vi "Get Channel Groups.vi"(7 "Settings(JSON)":string, 8 "error in":errorcluster, 9 "Channel Paths":string[](array[string]), 10 "Channel TypeNames":string[](array[string]), 11 "Channel JSONs":string[](array[string])) -> (0 "error out":errorcluster, 3 "ChannelGroups":T1, 5 "Settings(JSON)":string)   [LabVIEW 2026, in "Template Deployment Hooks.lvlib"]
uses:
  Template Deployment Hooks.lvlib
  Types/Channel Mode.ctl
  <vilib>/JDP Science/JSONtext/Next JSON Value.vi
  <vilib>/JDP Science/JSONtext/String Subset.vi
  <vilib>/JDP Science/JSONtext/support/Strip Quotes and Unescape.vi
  <vilib>/JDP Science/JSONtext/Parsing/Advance past next JSON Value (inlined COPY).vi
  <vilib>/JDP Science/JSONtext/support/Unescape JSON string.vi
  <vilib>/JDP Science/JSONtext/Parsing/Advance past whitespace.vi
  <vilib>/JDP Science/JSONtext/Parsing/Advance past String.vi
  <vilib>/JDP Science/JSONtext/Parsing/Advance past Number.vi
  <vilib>/JDP Science/JSONtext/Parsing/Advance past Line Ending.vi
  <vilib>/JDP Science/JSONtext/Parsing/Parse Full Path or Item Name.vi
  <vilib>/JDP Science/JSONtext/Parsing/Advance past Array.vi
  <vilib>/JDP Science/JSONtext/Parsing/Advance past Object.vi
  <vilib>/JDP Science/JSONtext/support/Error Cluster From Code.vi
  <vilib>/JDP Science/JSONtext/Offset/Find Item Locations by Path.vi
  <vilib>/JDP Science/JSONtext/Parsing/Advance past next JSON Value.vi
  <vilib>/JDP Science/JSONtext/JSONtext.lvlib
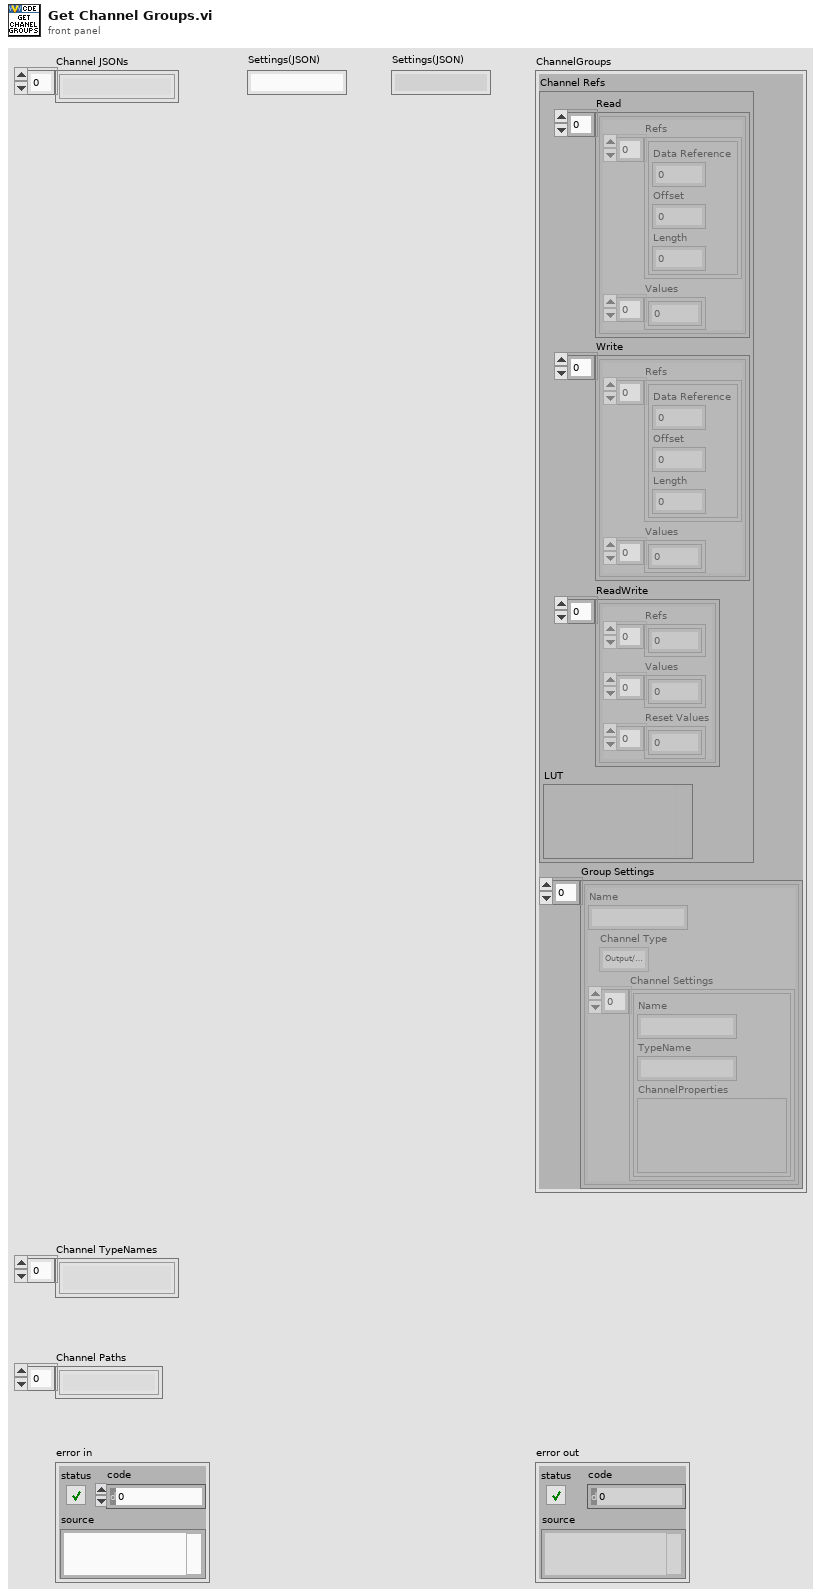
[diagram p1: front panel]
types:
  T1 = cluster{"Channel Refs":cluster{"Read":cluster{"Refs":cluster{"Data Reference":i32, "Offset":u64, "Length":u64}[], "Values":dbl[]}[], "Write":cluster{"Refs":cluster{"Data Reference":i32, "Offset":u64, "Length":u64}[], "Values":dbl[]}[], "ReadWrite":cluster{"Refs":i32[], "Values":dbl[], "Reset Values":dbl[]}[], "LUT":variant}, "Group Settings":cluster{"Name":string, "Channel Type":enum16{"Output/Write", "Input/Read", "Input/ReadWrite"}, "Channel Settings":cluster{"Name":string, "TypeName":string, "ChannelProperties":variant}[]}[]}
  T2 = typedef "Template Deployment Hooks.lvlib/Channel Mode.ctl" = enum16{"Output/Write", "Input/Read", "Input/ReadWrite"}
  T3 = cluster{"Group Name":string, "Channel Type":T2, "Channel DataReferences":i32[]}[]
  T4 = cluster{"Name":string, "Channel Type":enum16{"Output/Write", "Input/Read", "Input/ReadWrite"}, "Channel Settings":cluster{"Name":string, "TypeName":string, "ChannelProperties":variant}[]}[]
  T5 = cluster{"Name":string, "TypeName":string, "ChannelProperties":variant}
  T6 = cluster{"Group Name":string, "Channel Type":T2, "Channel Data References":i32[]}[]
  T7 = cluster{"Read":cluster{"Refs":cluster{"Data Reference":i32, "Offset":u64, "Length":u64}[], "Values":dbl[]}[], "Write":cluster{"Refs":cluster{"Data Reference":i32, "Offset":u64, "Length":u64}[], "Values":dbl[]}[], "ReadWrite":cluster{"Refs":i32[], "Values":dbl[], "Reset Values":dbl[]}[], "LUT":variant}
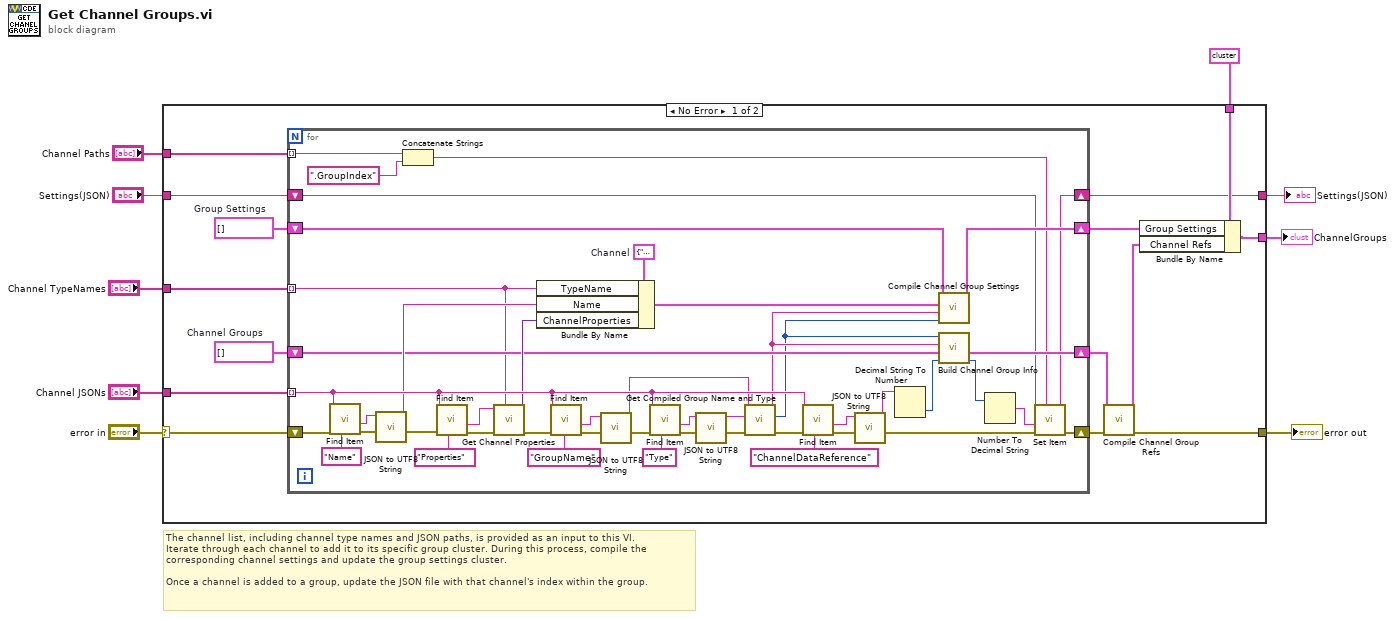
[diagram p0: block diagram]
diagram:
  # "The channel list, including channel type names and JSON paths, is provided as an input to this VI. \nIterate through each channel to add it to its specific group cluster. During this process, compile the corresponding channel settings and update the group settings cluster. \n\nOnce a channel is added to a group, update the JSON file with that channel's index within the group."
  n1 = case shown="No Error" "error in" {
    selector: "error in" -> [w23 w71]
    tunnel: [w24 w71] -> w8
    tunnel: "Channel JSONs" -> [w21 _]
    tunnel: "Channel TypeNames" -> [w20 _]
    tunnel: [w19 _] -> w5
    tunnel: T1 {"Channel Refs"={"Read"=[], "Write"=[], "ReadWrite"=[], "LUT"=variant}, "Group Settings"=[]} ("ChannelGroups") -> [w13 _]
    tunnel: "Channel Paths" -> [w12 _]
    tunnel: "Settings(JSON)" -> [w11 w70]
    tunnel: [w10 w70] -> w1
    frame No Error {
      w14 = T3 []  # Channel Groups
      w18 = T4 []  # Group Settings
      n2 = for {
        shift-right: [w58] -> w22
        shift-left: w23 -> [w69]
        tunnel: w21 -> [w52] mode=indexing
        tunnel: w20 -> [w32] mode=indexing
        shift-right: [w43] -> w16
        shift-left: w18 -> [w44]
        shift-right: [w39] -> w15
        shift-left: w14 -> [w38]
        tunnel: w12 -> [w29] mode=indexing
        shift-right: [w27] -> w10
        shift-left: w11 -> [w28]
        w48 = T5 {"Name"="", "TypeName"="", "ChannelProperties"=variant}  # Channel
        n3 = call <vilib>:"Find Item.vi"("$Path or Item Name"="Name", "error in (no error)"=w69, "JSON"=w52) -> ("error out"=w68:errorcluster, "<JSON>"=w51:string)  [unwired: 5 in, 2 out]
        n4 = call <vilib>:"JSON to UTF8 String.vi"("error in (no error)"=w68, "JSON"=w51) -> ("error out"=w67:errorcluster, "<UTF8>String"=w45:string)  [unwired: 8 in]
        n5 = Concatenate Strings(w29, ".GroupIndex" ("string")) -> (w26:string)
        n6 = call <vilib>:"Find Item.vi"("$Path or Item Name"="Properties", "error in (no error)"=w67, "JSON"=w52) -> ("error out"=w62:errorcluster, "<JSON>"=w42:string)  [unwired: 5 in, 2 out]
        n7 = call "Get Channel Properties.vi"("TypeName"=w32, "error in"=w62, "JSON"=w42) -> ("error out"=w61:errorcluster, "Channel Properties"=w47:variant)  [unwired: 7 in]
        n8 = Bundle By Name(cluster=w48, "TypeName"=w32, "Name"=w45, "ChannelProperties"=w47) -> (w46:T5)
        n9 = call <vilib>:"Find Item.vi"("$Path or Item Name"="GroupName", "error in (no error)"=w61, "JSON"=w52) -> ("error out"=w66:errorcluster, "<JSON>"=w49:string)  [unwired: 5 in, 2 out]
        n10 = call <vilib>:"JSON to UTF8 String.vi"("error in (no error)"=w66, "JSON"=w49) -> ("error out"=w65:errorcluster, "<UTF8>String"=w40:string)  [unwired: 8 in]
        n11 = call <vilib>:"Find Item.vi"("$Path or Item Name"="Type", "error in (no error)"=w65, "JSON"=w52) -> ("error out"=w64:errorcluster, "<JSON>"=w50:string)  [unwired: 5 in, 2 out]
        n12 = call <vilib>:"JSON to UTF8 String.vi"("error in (no error)"=w64, "JSON"=w50) -> ("error out"=w63:errorcluster, "<UTF8>String"=w41:string)  [unwired: 8 in]
        n13 = call "Get Compiled Group Name and Type.vi"("Channel Type"=w41, "Group Name"=w40) -> ("Group Type"=w35:T2, "Computed Group Name"=w37:string)  [unwired: 8 in]
        n14 = call <vilib>:"Find Item.vi"("$Path or Item Name"="ChannelDataReference", "error in (no error)"=w63, "JSON"=w52) -> ("error out"=w60:errorcluster, "<JSON>"=w34:string)  [unwired: 5 in, 2 out]
        n15 = call <vilib>:"JSON to UTF8 String.vi"("error in (no error)"=w60, "JSON"=w34) -> ("error out"=w59:errorcluster, "<UTF8>String"=w33:string)  [unwired: 8 in]
        n16 = Decimal String To Number(string=w33) -> (number=w36:i32)  [unwired: 2 in, 1 out]
        n17 = call "Compile Channel Group Settings.vi"("Channel Type"=w35, "Group Name"=w37, "ChannelSettings"=w46, "Group Settings"=w44) -> ("Group Settings"=w43:T4)  [unwired: 7 in]
        n18 = call "Build Channel Group Info.vi"("Channel Data Reference"=w36, "Channel Groups in"=w38, "Group Name"=w37, "Channel Type"=w35) -> ("Group Index"=w31:i32, "Channel Groups out"=w39:T6)  [unwired: 6 in]
        n19 = Number To Decimal String(number=w31) -> (decimal integer string=w30:string)  [unwired: 1 in]
        n20 = call <vilib>:"Set Item.vi"("$Path or Item Name"=w26, "error in (no error)"=w59, "JSON to Insert"=w30, "JSON"=w28) -> ("error out"=w58:errorcluster, "<JSON>"=w27:string)  [unwired: 4 in, 1 out]
      }
      n21 = call "Compile Channel Group Refs.vi"("error in"=w22, "Channel Groups in"=w15) -> ("error out"=w24:errorcluster, "CompiledChannelGroupings"=w17:T7)  [unwired: 8 in]
      n22 = Bundle By Name(cluster=w13, "Group Settings"=w16, "Channel Refs"=w17) -> (w19:T1)
    }
    frame Error {
    }
  }
  "error out" <- w8
  "ChannelGroups" <- w5
  "Settings(JSON)" <- w1
